vi "畫橢圓.vi"(8 "error in (no error)":errorcluster, 9 "Color":u32(colorbox)=16711680, 10 "Ellipse":T2 {"Minor Axis"."Point 2"."Y" format="%.2f"; "Minor Axis"."Point 2"."X" format="%.2f"; "Minor Axis"."Point 1"."Y" format="%.2f"; "Minor Axis"."Point 1"."X" format="%.2f"; "Major Axis"."Point 2"."Y" format="%.2f"; "Major Axis"."Point 2"."X" format="%.2f"; "Major Axis"."Point 1"."Y" format="%.2f"; "Major Axis"."Point 1"."X" format="%.2f"; "Center"."Y" format="%.2f"; "Center"."X" format="%.2f"}, 11 "Image In":T1) -> (0 "error out":errorcluster, 3 "Image":T1(plugin-control))   [LabVIEW 2015]
uses:
  <vilib>/vision/Image Controls.llb/IMAQ Image.ctl
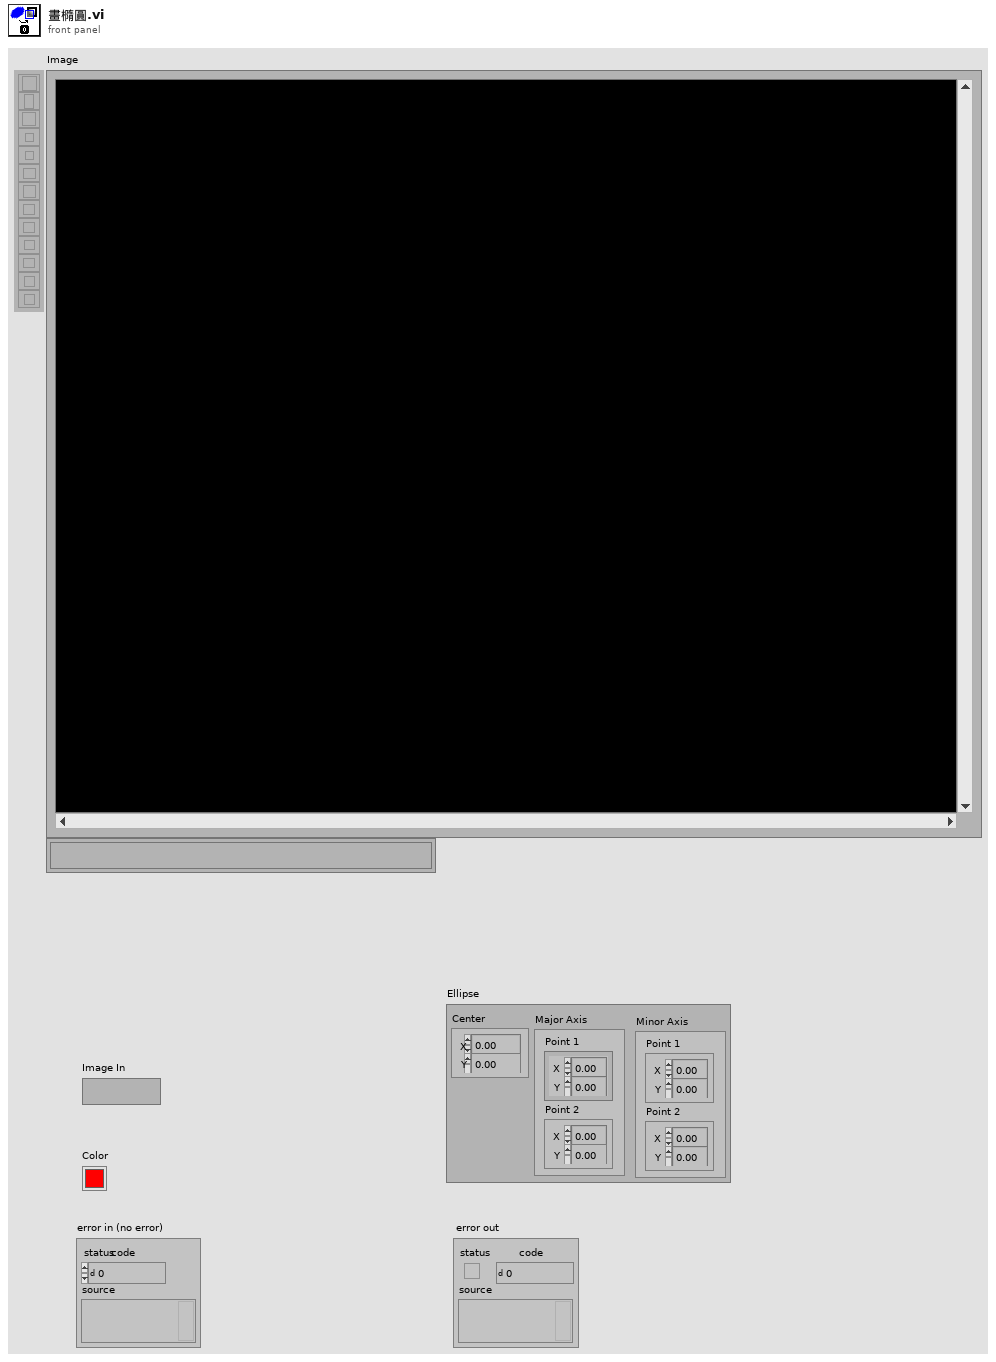
[diagram p1: front panel]
types:
  T1 = typedef "IMAQ Image.ctl" = refnum<image>
  T2 = cluster{"Center":cluster{"X":sgl, "Y":sgl}, "Major Axis":cluster{"Point 1":cluster{"X":sgl, "Y":sgl}, "Point 2":cluster{"X":sgl, "Y":sgl}}, "Minor Axis":cluster{"Point 1":cluster{"X":sgl, "Y":sgl}, "Point 2":cluster{"X":sgl, "Y":sgl}}}
  T3 = cluster{"Point 1":cluster{"X":sgl, "Y":sgl}, "Point 2":cluster{"X":sgl, "Y":sgl}}
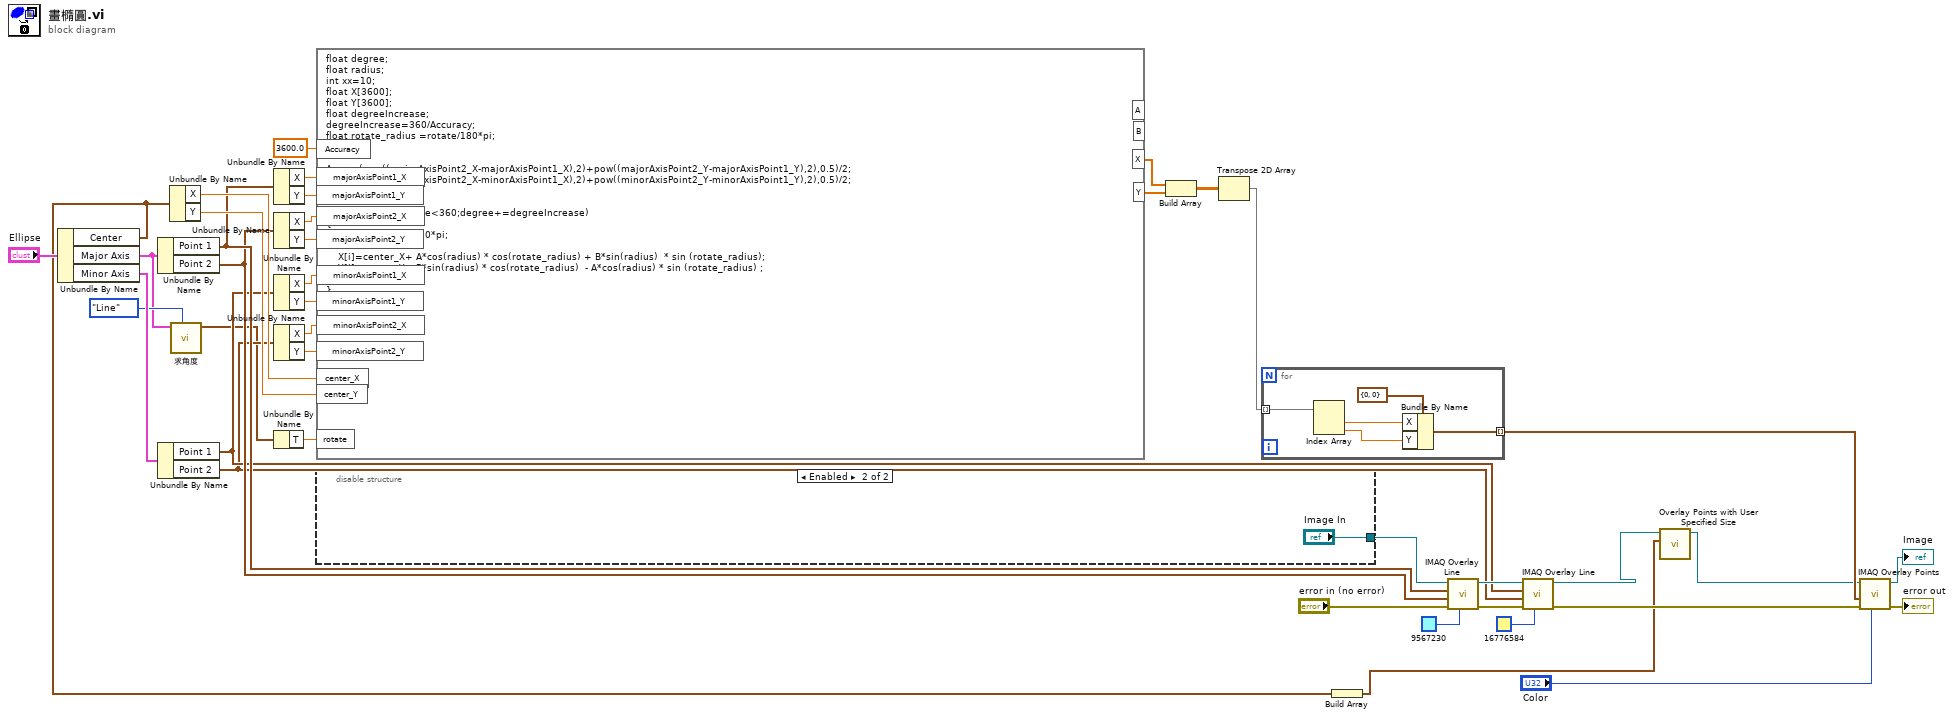
[diagram p0: block diagram]
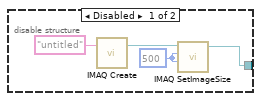
[diagram p2: hidden frame]
diagram:
  n1 = Unbundle By Name("Ellipse") -> ("Center"=w4:cluster{"X":sgl, "Y":sgl}, "Major Axis"=w16:T3, "Minor Axis"=w36:T3)
  n2 = Unbundle By Name(w16) -> ("Point 1"=w24:cluster{"X":sgl, "Y":sgl}, "Point 2"=w21:cluster{"X":sgl, "Y":sgl})
  n3 = Unbundle By Name(w36) -> ("Point 1"=w20:cluster{"X":sgl, "Y":sgl}, "Point 2"=w19:cluster{"X":sgl, "Y":sgl})
  n4 = Unbundle By Name(w4) -> ("X"=w31:sgl, "Y"=w30:sgl)
  n5 = call "求角度.vi"("Line form"=enum16{"Line", "Two Point"}."Line", "Line"=w16) -> ("Line Data"=w8:cluster{"X":sgl, "Y":sgl, "T":sgl})  [unwired: 9 in]
  n6 = Unbundle By Name(w24) -> ("X"=w40:sgl, "Y"=w39:sgl)
  n7 = Unbundle By Name(w21) -> ("X"=w38:sgl, "Y"=w37:sgl)
  n8 = Unbundle By Name(w20) -> ("X"=w35:sgl, "Y"=w34:sgl)
  n9 = Unbundle By Name(w19) -> ("X"=w33:sgl, "Y"=w32:sgl)
  n10 = Unbundle By Name(w8) -> ("T"=w7:sgl)
  n11 = formula code="float degree;\nfloat radius;\nint xx=10;\nfloat X[3600];\nfloat Y[3600];\nfloat degreeIncrease;\ndegreeIncrease=360/Accuracy;\nfloat rotate_radius =rotate/180*pi;\nint i=0;\n\nA=pow(pow((majorAxisPoint2_X-majorAxisPoint1_X),2)+pow((majorAxisPoint2_Y-majorAxisPoint1_Y),2),0.5)/2;\nB=pow(pow((minorAxisPoint2_X-minorAxisPoint1_X),2)+pow((minorAxisPoint2_Y-minorAxisPoint1_Y),2),0.5)/2;\n\n\nfor (degree=0;degree<360;degree+=degreeIncrease)\n{\n    radius=degree/180*pi;\n\n    X[i]=center_X+ A*cos(radius) * cos(rotate_radius) + B*sin(radius)  * sin (rotate_radius);\n    Y[i]=center_Y+ B*sin(radius) * cos(rotate_radius)  - A*cos(radius) * sin (rotate_radius) ;\n    i++;\n}"("majorAxisPoint1_X"=w40, "majorAxisPoint1_Y"=w39, "majorAxisPoint2_X"=w38, "majorAxisPoint2_Y"=w37, "minorAxisPoint1_X"=w35, "minorAxisPoint1_Y"=w34, "minorAxisPoint2_X"=w33, "minorAxisPoint2_Y"=w32, "center_X"=w31, "center_Y"=w30, "rotate"=w7, "Accuracy"=3600.0 ("input variable")) -> ("X"=w15:dbl[], "Y"=w14:dbl[])  [unwired: 2 out]
  n12 = disable-structure shown="Enabled" {
    disable-tunnel: [w41 "Image In"] -> w25
    frame Disabled {
      w42 = 500 ("X Resolution")
      n13 = call "IMAQ Create"("Image Name"="untitled") -> ("New Image"=w43:T1)  [unwired: 4 in, 1 out]
      n14 = call "IMAQ SetImageSize"("Y Resolution"=w42, "X Resolution"=w42, "Image"=w43) -> ("Image Out"=w41:T1)  [unwired: 2 in, 1 out]
    }
    frame Enabled {
    }
  }
  n15 = Build Array(w15, w14) -> (w29:dbl[][])
  n16 = Transpose 2D Array(2D array=w29) -> (transposed array=w1:dbl[][])
  n17 = for {
    tunnel: w1 -> [w50] mode=indexing
    tunnel: [w49] -> w27 mode=indexing
    n18 = Index Array(array=w50) -> (element #1=w47:dbl, element #2=w46:dbl)  [unwired: 2 in]
    n19 = Bundle By Name(cluster=cluster{"X":i32, "Y":i32} {"X"=0, "Y"=0}, "X"=w47, "Y"=w46) -> (w49:cluster{"X":i32, "Y":i32})
  }
  n20 = Build Array(w4) -> (w3:cluster{"X":sgl, "Y":sgl}[])
  n21 = call "IMAQ Overlay Line"("Color"=u32 9567230, "error in (no error)"="error in (no error)", "End Point"=w21, "Start Point"=w24, "Image"=w25) -> ("error out"=w11:errorcluster, "Image Out"=w26:T1)  [unwired: 5 in]
  n22 = call "IMAQ Overlay Line"("Color"=u32 16776584, "error in (no error)"=w11, "End Point"=w19, "Start Point"=w20, "Image"=w26) -> ("error out"=w10:errorcluster, "Image Out"=w6:T1)  [unwired: 5 in]
  n23 = call "Overlay Points with User Specified Size.vi"("Points"=w3, "Image In"=w6) -> ("Image Out"=w5:T1)  [unwired: 8 in, 1 out]
  n24 = call "IMAQ Overlay Points"("Color"="Color", "error in (no error)"=w10, "Array of Points"=w27, "Image"=w5) -> ("error out"=→"error out":errorcluster, "Image Out"=→"Image":T1)  [unwired: 6 in]
